vi "analog_voltage_update.vi"(8 "error in (no error)":errorcluster, 10 "ExperimentVariables (in)":refnum<class "ExperimentVariables.lvclass">, 11 "Analog Output Parameters":T1={"Enable Analog Out?"=TRUE, "Physical Channel"="PXI1Slot2/ao0", "Trigger Source"="/PXI1Slot6/do/StartTrigger", "Minimum Value"=-10.0, "Maximum Value"=10.0, "Samples per second"=10000.0, "Samples per Waveform"=20000.0, "Analog Output Channels"=[{"Analog Output Equation"="7*(1-spike((t-0.02)*1000)/200)", "Frequency"=0.0, "Amplitude"=0.0}]} {"Maximum Value" format="%0.2f"; "Minimum Value" format="%0.2f"}) -> (0 "error out":errorcluster, 2 "ExperimentVariables":refnum<class "ExperimentVariables.lvclass">, 3 "analog output DAQmx task":refnum<k21>)   [LabVIEW 2011]
doc: "I. Description:\nThis example demonstrates how to output a single Voltage Update (Sample) to an Analog Output Channel.\n\nII. Instructions for Running:\n1. Select the Physical Channel to correspond to where your signal is output on the DAQ device.\n2. Enter the Minimum and Maximum Voltage Ranges\nNote: Use the Acq One Sample example to verify you are generating the correct output on the DAQ device\n\nIII. Block Diagram Steps:\n1. Create an Analog Output Voltage Channel\n2. Use the Write VI to Output 1 Sample to 1 Channel on the Data\nAcquisition Card. \n3. Call the Clear Task VI to clear the Task.\n4. Use the popup dialog box to display an error if any. \n\nIV. I/O Connections Overview:\nMake sure your signal output terminal matches the Physical Channel I/O Control. For further connection information, refer to your hardware reference manual."
uses:
  ExperimentVariables/ExperimentVariables.lvclass
  <vilib>/DAQmx/write.llb/DAQmx Write (Analog 1D Wfm NChan NSamp).vi
  <vilib>/DAQmx/create/channels.llb/DAQmx Create Channel (AO-Voltage-Basic).vi
  <vilib>/DAQmx/configure/timing.llb/DAQmx Timing (Sample Clock).vi
  <vilib>/DAQmx/configure/trigger.llb/DAQmx Start Trigger (Digital Edge).vi
  <vilib>/DAQmx/miscellaneous.llb/DAQmx Fill In Error Info.vi
  <vilib>/measure/NI_MAPro.lvlib
  <vilib>/gmath/NI_Gmath.lvlib
panel:
  out "Waveform Graph":waveform(dbl)[](graph)
  # "If 't' is not specified in the variables or paramaters, it will be used here as time in seconds.\nNote, analog output will only continue until the digital pulse output is done, or until Samples per Waveform runs out, whichever comes first."
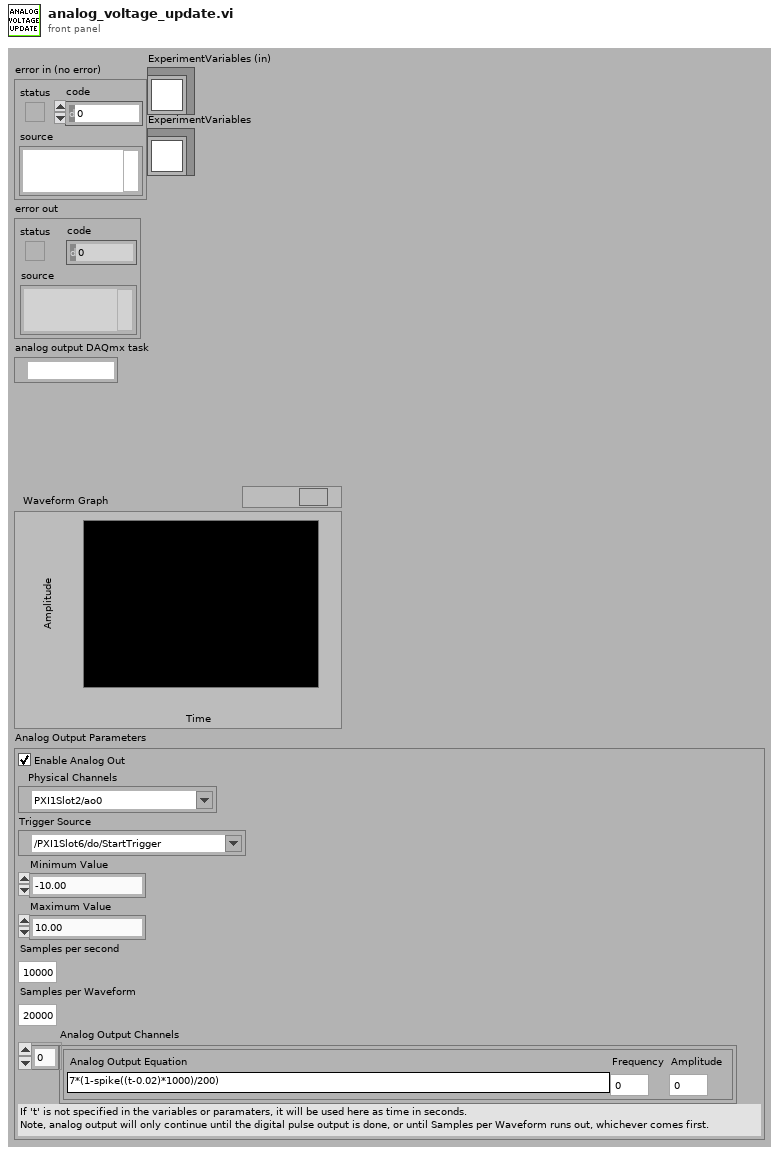
[diagram p1: front panel]
types:
  T1 = cluster{"Enable Analog Out?":bool, "Physical Channel":tag, "Trigger Source":tag, "Minimum Value":dbl, "Maximum Value":dbl, "Samples per second":dbl, "Samples per Waveform":dbl, "Analog Output Channels":cluster{"Analog Output Equation":string, "Frequency":dbl, "Amplitude":dbl}[]}
  T2 = cluster{"Analog Output Equation":string, "Frequency":dbl, "Amplitude":dbl}[]
  T3 = cluster{"Samples per second":dbl, "Samples per Waveform":dbl}
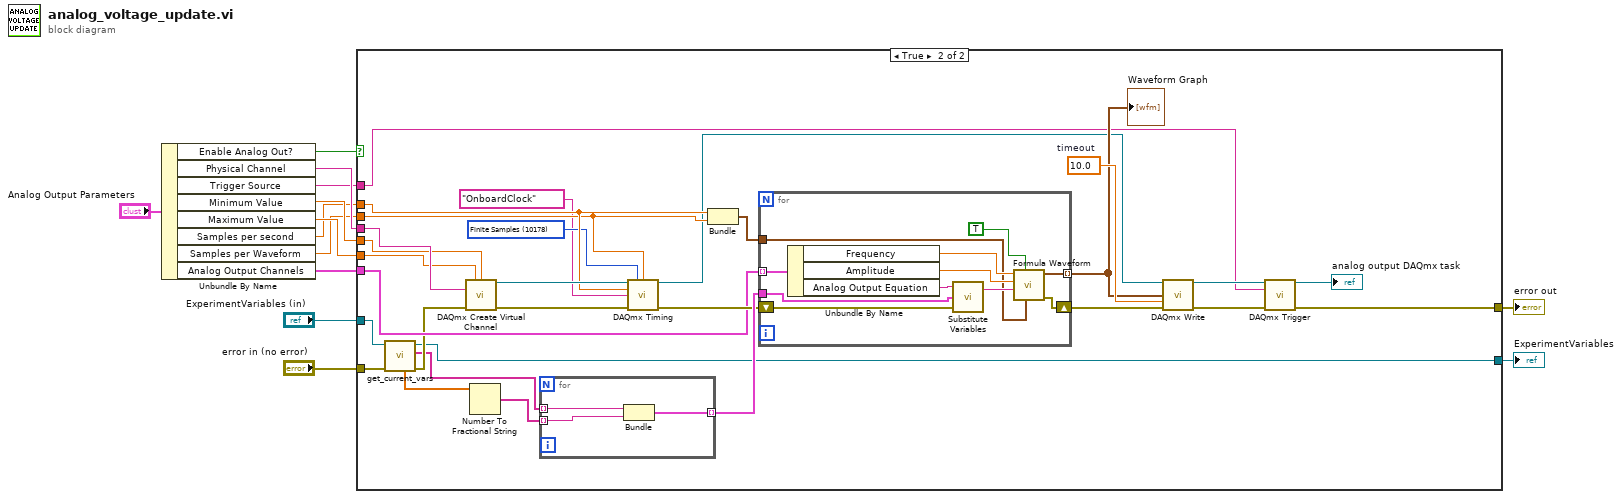
[diagram p0: block diagram]
diagram:
  n1 = Unbundle By Name("Analog Output Parameters") -> ("Enable Analog Out?"=w8:bool, "Physical Channel"=w11:tag, "Trigger Source"=w3:tag, "Minimum Value"=w9:dbl, "Maximum Value"=w10:dbl, "Samples per second"=w7:dbl, "Samples per Waveform"=w6:dbl, "Analog Output Channels"=w4:T2)
  n2 = case shown="True" w8 {
    tunnel: "error in (no error)" -> [w15 w21]
    tunnel: [w15 w33] -> w12
    tunnel: w11 -> [_ w44]
    tunnel: w10 -> [_ w43]
    tunnel: w9 -> [_ w42]
    tunnel: w7 -> [_ w37]
    tunnel: w6 -> [_ w31]
    tunnel: w4 -> [_ w23]
    tunnel: w3 -> [_ w22]
    tunnel: "ExperimentVariables (in)" -> [w14 w17]
    tunnel: [w14 w16] -> w1
    frame False {
    }
    frame True {
      w32 = 10178 items=["Finite Samples"=10178, "Continuous Samples"=10123, "Hardware Timed Single Point"=12522] ("sample mode")
      w27 = 10.0  # timeout
      n3 = call-dynamic "get_current_vars.vi"("error in (no error)"=w21, "ExperimentVariables in"=w17) -> ("error out"=w20:errorcluster, "variables and parameter names"=w18:string[], "ExperimentVariables out"=w16:refnum<class "ExperimentVariables.lvclass">, "current variable and parameter values"=w19:dbl[])  [unwired: 4 in, 2 out]
      n4 = call-poly <vilib>:"DAQmx Create Virtual Channel.vi"("maximum value"=w43, "minimum value"=w42, "physical channels"=w44, "error in"=w20) -> ("task out"=w38:refnum<k21>, "error out"=w36:errorcluster)  [unwired: 10 in]
      n5 = Number To Fractional String(number=w19) -> (F-format string=w41:string[])  [unwired: 3 in]
      n6 = for {
        tunnel: w18 -> [w58] mode=indexing
        tunnel: w41 -> [w57] mode=indexing
        tunnel: [w56] -> w40 mode=indexing
        n7 = Bundle(w58, w57) -> (w56:cluster{string, string})  [unwired: 1 in]
      }
      n8 = call-poly <vilib>:"DAQmx Timing.vi"("task/channels in"=w38, "sample mode"=w32, "samples per channel"=w31, "rate"=w37, "source"=tag "OnboardClock", "error in"=w36) -> ("task out"=w25:refnum<k21>, "error out"=w29:errorcluster)  [unwired: 8 in]
      n9 = Bundle("Samples per second"=w37, "Samples per Waveform"=w31) -> (w39:T3)  [unwired: 1 in]
      n10 = for {
        tunnel: w23 -> [w55] mode=indexing
        tunnel: w40 -> [w54]
        shift-right: [w50] -> w28
        shift-left: w29 -> [w51]
        tunnel: w39 -> [w46]
        tunnel: [w45] -> w26 mode=indexing
        n11 = Unbundle By Name(w55) -> ("Frequency"=w49:dbl, "Amplitude"=w48:dbl, "Analog Output Equation"=w53:string)
        n12 = call <vilib>:"Substitute Variables.vi"("error in (no error)"=w51, "Substitution Rules"=w54, "original formula"=w53) -> ("formula after substitution"=w52:string)  [unwired: 1 out]
        n13 = call <vilib>:"Formula Waveform.vi"("sampling info"=w46, "reset signal"=TRUE, "formula"=w52, "amplitude"=w48, "frequency"=w49) -> ("error out"=w50:errorcluster, "signal out"=w45:waveform(dbl))  [unwired: 5 in]
      }
      "Waveform Graph" <- w26
      n14 = call-poly <vilib>:"DAQmx Write.vi"("task/channels in"=w25, "data"=w26, "timeout"=w27, "error in"=w28) -> ("task out"=w35:refnum<k21>, "error out"=w24:errorcluster)  [unwired: 9 in, 1 out]
      n15 = call-poly <vilib>:"DAQmx Trigger.vi"("task/channels in"=w35, "source"=w22, "error in"=w24) -> ("task out"=→"analog output DAQmx task":refnum<k21>, "error out"=w33:errorcluster)  [unwired: 11 in]
    }
  }
  "error out" <- w12
  "ExperimentVariables" <- w1
